vi "FORM_BORD.vi"(0 "VISA IN":refnum<visa-resource-name>, 5 "error in":errorcluster, 7 "Border":string(combo)="NORM") -> (14 "VISA Out":refnum<visa-resource-name>, 19 "error out":errorcluster)   [LabVIEW 2018, in "PNA-X.lvlib"]
doc: "FORMat:BORDer <char> \n(Read-Write) Set the byte order used for GPIB data transfer. Some computers read data from the \nanalyzer in the reverse order. This command is only implemented if FORMAT:DATA is set to \n:REAL. If FORMAT:DATA is set to :ASCII, the swapped command is ignored. \nParameters \n<char> Choose from: \nNORMal - Use when your controller is anything other than an IBM compatible \ncomputers \nSWAPped - for IBM compatible computers \nNote: Use NORMal if you are using drivers like VISA or development \nenvironments like VEE, LabView, or T&M Tool kit. \nExamples FORM:BORD SWAP \nformat:border normal \nQuery Syntax FORMat:BORDer? \nReturn Type Character \n1602\n\nDefault Normal \nFORMat[:DATA] <char> \n(Read-Write) Sets the data format for data transfers. \nTo transfer measurement data, use CALC:DATA. \nTo transfer Cal Set data, use \nTo transfer Source Power correction data, use \nSOURce:POWer:CORRection:COLLect:TABLe:DATA \nSOURce:POWer:CORRection:COLLect:TABLe:FREQuency"
uses:
  PNA-X.lvlib
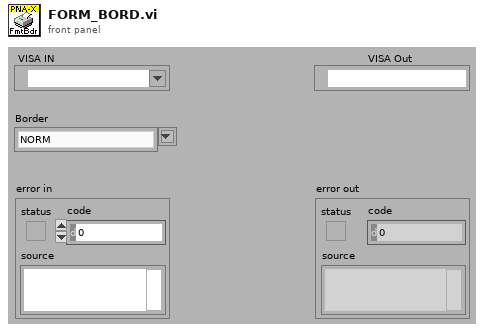
[diagram p1: front panel]
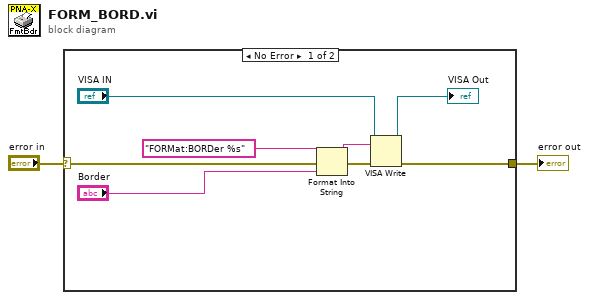
[diagram p0: block diagram]
diagram:
  n1 = case shown="No Error" "error in" {
    selector: "error in" -> [w10 w11]
    tunnel: [w5 w11] -> w1
    frame No Error {
      n2 = Format Into String(format string="FORMat:BORDer %s" ("Cmdline"), error in=w10, "Border") -> (resulting string=w8:string, error out=w9:errorcluster)  [unwired: 1 in]
      n3 = VISA Write(VISA resource name="VISA IN", write buffer=w8, error in (no error)=w9) -> (VISA resource name out=→"VISA Out":refnum<visa-resource-name>, error out=w5:errorcluster)  [unwired: 1 out]
    }
    frame Error {
    }
  }
  "error out" <- w1
